vi "Calculate Replace Index.vi"(10 "Seqno":u8, 11 "Block Upload Transfer in":refnum<class "Block Upload Sub-Block Transfer.lvclass">) -> (3 "Replace Index":u8)   [LabVIEW 2020, in "CANopen.lvlib" / "SDO Manager.lvlib" / "Block Upload Sub-Block Transfer.lvclass"]
uses:
  Block Upload Sub-Block Transfer.lvclass
  Block Upload Sub-Block Transfer.lvclass/Block Upload Sub-Block Transfer.ctl
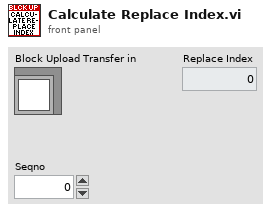
[diagram p1: front panel]
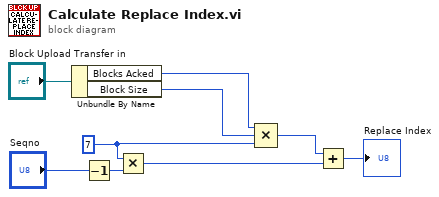
[diagram p0: block diagram]
diagram:
  w8 = u8 7 ("x")
  n1 = Unbundle By Name("Block Upload Transfer in") -> ("Blocks Acked"=w3:u8, "Block Size"=w4:u8)
  n2 = Decrement(x="Seqno") -> (x-1=w5:u8)
  n3 = Multiply(x=w8, y=w5) -> (x*y=w6:u8)
  n4 = Compound Arithmetic op=MULTIPLY(w3, w4, w8) -> (w7:u8)
  n5 = Add(x=w7, y=w6) -> (x+y=→"Replace Index":u8)
